vi "Read RawData.vi"(8 "error in (no error)":errorcluster, 9 "WCM_max_value":bool, 10 "# of scans":i32, 11 "Emulate in":refnum<class "Emulate.lvclass">) -> (0 "error out":errorcluster, 1 "Channel II":sgl[][](array[numeric]), 2 "Channel I":sgl[][](array[numeric]), 3 "Emulate out":refnum<class "Emulate.lvclass">, 4 "WCM_values":sgl[](array[numeric]))   [LabVIEW 2015, in "Emulate.lvclass"]
uses:
  Emulate.lvclass
  dependecies/globalVarII.vi
panel:
  out "Waveform Graph 2":i32[][](graph)
  out "Waveform Graph":i32[][](graph)
  in  "A":dbl=15000.0
  in  "pos":dbl=550.0 format="%#_13g"
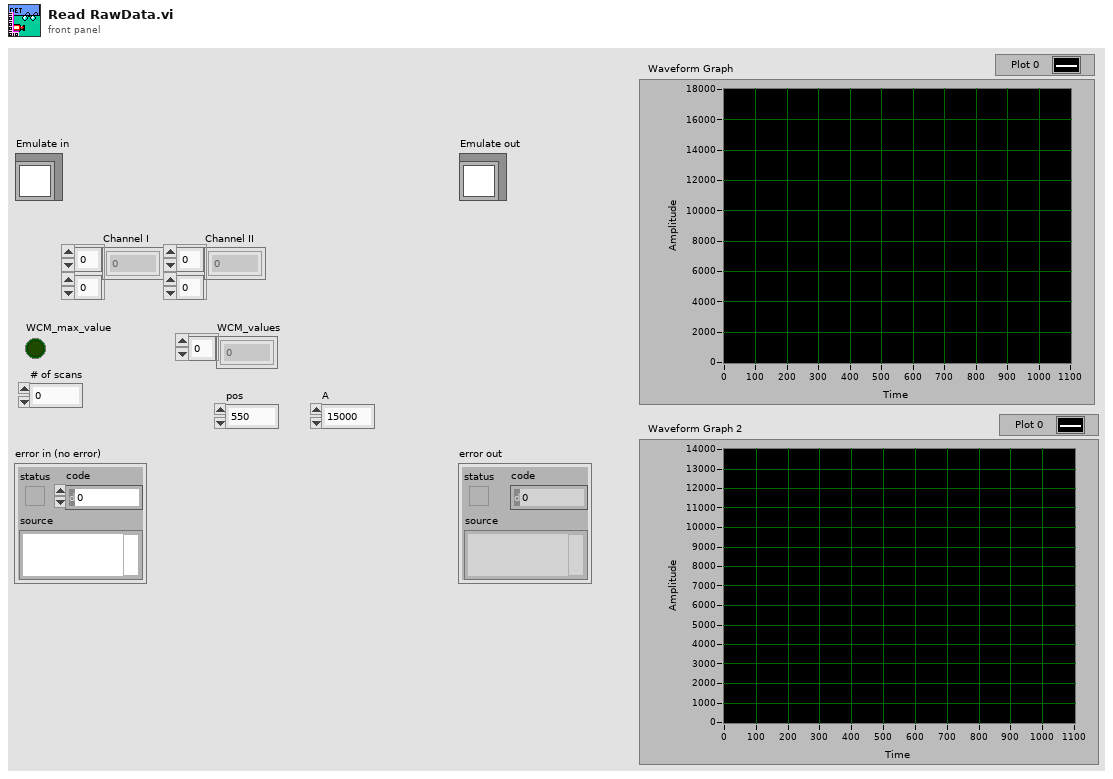
[diagram p1: front panel]
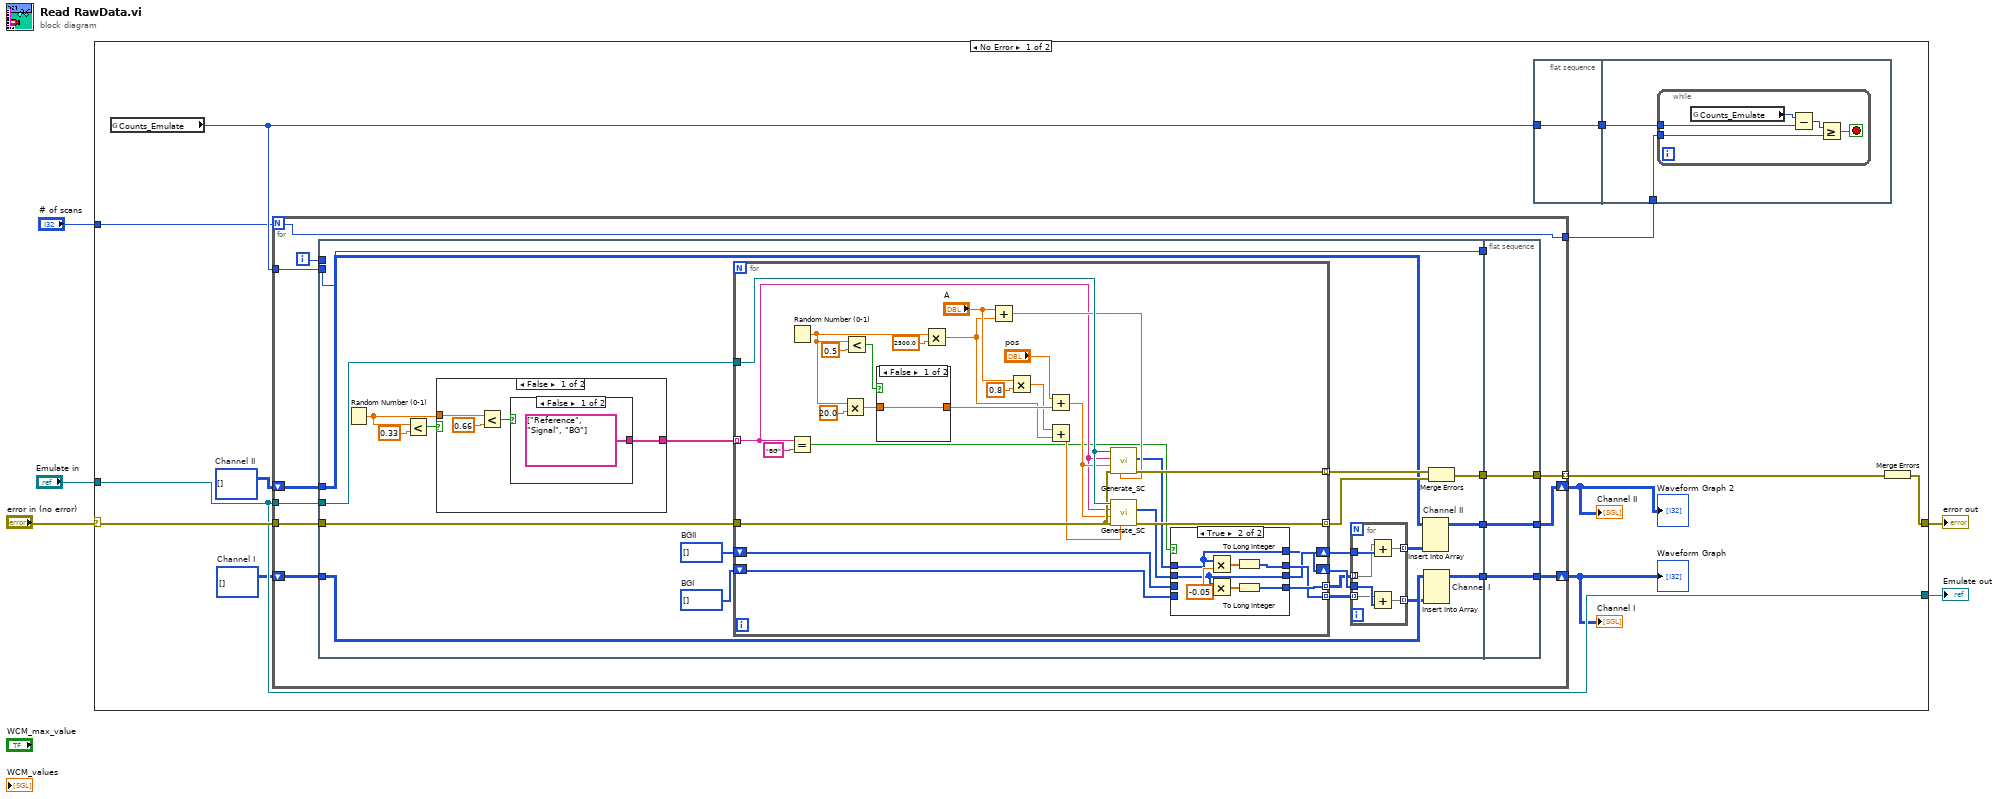
[diagram p0: block diagram]
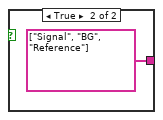
[diagram p2: hidden frame]
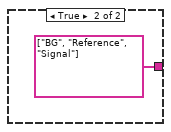
[diagram p3: hidden frame]
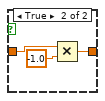
[diagram p5: hidden frame]
diagram:
  n1 = case shown="No Error" "error in (no error)" {
    selector: "error in (no error)" -> [w17 w124]
    tunnel: [w15 w124] -> w4
    tunnel: [w14 w123] -> w3
    tunnel: "Emulate in" -> [w14 w123]
    tunnel: "# of scans" -> [w9 _]
    frame No Error {
      w12 = i32[][] []  # Channel II
      w13 = i32[][] []  # Channel I
      n2 = global read "globalVarII.vi" "Counts_Emulate"() -> (w11:i64)
      n3 = for {
        N: w9 -> [w26]
        tunnel: w14 -> [w39]
        tunnel: w17 -> [w38]
        tunnel: [w37] -> w16 mode=indexing
        shift-right: [w36] -> w8
        shift-left: w13 -> [w35]
        shift-right: [w34] -> w7
        shift-left: w12 -> [w33]
        tunnel: w11 -> [w28]
        tunnel: [w26] -> w6
        i -> [w27]
        n4 = flat-sequence {
          tunnel: w39 -> [w57]
          tunnel: w38 -> [w56]
          tunnel: w35 -> [w51]
          tunnel: w33 -> [w49]
          tunnel: [w53] -> w32
          tunnel: [w52] -> w31
          tunnel: [w50] -> w30
          tunnel: [w48] -> w29
          tunnel: w28 -> [w48]
          tunnel: w27 -> [_]
          tunnel: [w120] -> w34
          tunnel: [w121] -> w36
          tunnel: [w122] -> w37
          tunnel: w32 -> [w122]
          tunnel: w31 -> [w121]
          tunnel: w30 -> [w120]
          tunnel: w29 -> [_]
          frame #0 {
            w47 = i32[] []  # BGII
            w46 = i32[] []  # BGI
            n5 = Random Number (0-1)() -> (number: 0 to 1=w58:dbl)
            n6 = Less?(x=w58, y=0.33) -> (x < y?=w59:bool)
            n7 = case shown="False" w59 {
              tunnel: [w68 string[] ["BG", "Reference", "Signal"] ("appended array")] -> w61
              tunnel: w58 -> [w71 _]
              frame False {
                n8 = Less?(x=w71, y=0.66) -> (x < y?=w69:bool)
                n9 = case shown="False" w69 {
                  tunnel: [string[] ["Reference", "Signal", "BG"] ("appended array") string[] ["Signal", "BG", "Reference"] ("appended array")] -> w68
                  frame False {
                  }
                  frame True {
                  }
                }
              }
              frame True {
              }
            }
            n10 = for {
              tunnel: w61 -> [w85] mode=indexing
              tunnel: w57 -> [w104]
              tunnel: w56 -> [w103]
              tunnel: [w102] -> w54 mode=indexing
              tunnel: [w101] -> w55 mode=indexing
              shift-right: [w80] -> w42
              shift-left: w47 -> [w79]
              shift-right: [w77] -> w45
              shift-left: w46 -> [w78]
              tunnel: [w82] -> w41 mode=indexing
              tunnel: [w81] -> w40 mode=indexing
              n11 = Random Number (0-1)() -> (number: 0 to 1=w93:dbl)
              n12 = Equal?(x=w85, y="BG") -> (x = y?=w83:bool)
              n13 = Multiply(x=w93, y=20.0) -> (x*y=w94:dbl)
              n14 = Less?(x=w93, y=0.5) -> (x < y?=w95:bool)
              n15 = case shown="False" w95 {
                tunnel: [w116 w117] -> w96
                tunnel: w94 -> [w116 w119]
                frame False {
                }
                frame True {
                  n16 = Multiply(x=w119, y=-1.0) -> (x*y=w117:dbl)
                }
              }
              n17 = Multiply(x=w93, y=2500.0) -> (x*y=w87:dbl)
              n18 = Add(x="A", y=w87) -> (x+y=w91:dbl)
              n19 = Multiply(x="A", y=0.8) -> (x*y=w88:dbl)
              n20 = Add(x="pos", y=w96) -> (x+y=w97:dbl)
              n21 = Add(x=w88, y=w87) -> (x+y=w86:dbl)
              n22 = call "Generate_SC.vi"("A"=w91, "error in (no error)"=w103, "pos"=w97, "Type of signal"=w85, "Emulate in"=w104) -> ("error out"=w101:errorcluster, "SC output"=w76:i32[])  [unwired: 4 in, 1 out]
              n23 = call "Generate_SC.vi"("A"=w86, "error in (no error)"=w103, "pos"=w97, "Type of signal"=w85, "Emulate in"=w104) -> ("error out"=w102:errorcluster, "SC output"=w75:i32[])  [unwired: 4 in, 1 out]
              n24 = case shown="True" w83 {
                tunnel: [w105 w111] -> w82
                tunnel: [w106 w112] -> w81
                tunnel: [w108 w109] -> w80
                tunnel: w79 -> [w108 _]
                tunnel: w78 -> [w107 _]
                tunnel: [w107 w110] -> w77
                tunnel: w76 -> [w106 w110]
                tunnel: w75 -> [w105 w109]
                frame False {
                }
                frame True {
                  w113 = -0.05
                  n25 = Multiply(x=w110, y=w113) -> (x*y=w115:dbl[])
                  n26 = Multiply(x=w109, y=w113) -> (x*y=w114:dbl[])
                  n27 = To Long Integer(number=w115) -> (32bit integer=w112:i32[])
                  n28 = To Long Integer(number=w114) -> (32bit integer=w111:i32[])
                }
              }
            }
            n29 = for {
              tunnel: w45 -> [w67]
              tunnel: [w66] -> w44 mode=indexing
              tunnel: [w65] -> w43 mode=indexing
              tunnel: w42 -> [w64]
              tunnel: w41 -> [w63] mode=indexing
              tunnel: w40 -> [w62] mode=indexing
              n30 = Add(x=w63, y=w64) -> (x+y=w65:i32[])
              n31 = Add(x=w62, y=w67) -> (x+y=w66:i32[])
            }
            n32 = Insert Into Array "Channel II"(array=w49, new element=w43) -> (w50:i32[][])  [unwired: 2 in]
            n33 = Insert Into Array "Channel I"(array=w51, new element=w44) -> (w52:i32[][])  [unwired: 2 in]
            n34 = Merge Errors(w55, w54) -> (w53:errorcluster)
          }
          frame #1 {
          }
        }
      }
      "Channel I" <- w8
      "Channel II" <- w7
      "Waveform Graph" <- w8
      "Waveform Graph 2" <- w7
      n35 = flat-sequence {
        tunnel: w11 -> [w18]
        tunnel: [w18] -> w10
        tunnel: w10 -> [w20]
        tunnel: w6 -> [w19]
        frame #0 {
        }
        frame #1 {
          n36 = while {
            tunnel: w20 -> [w23]
            tunnel: w19 -> [w21]
            stop <- w25 stop-if-true
            n37 = global read "globalVarII.vi" "Counts_Emulate"() -> (w24:i64)
            n38 = Subtract(x=w24, y=w23) -> (x-y=w22:i64)
            n39 = Greater Or Equal?(x=w22, y=w21) -> (x >= y?=w25:bool)
          }
        }
      }
      n40 = Merge Errors(w16) -> (w15:errorcluster)
    }
    frame Error {
    }
  }
  "error out" <- w4
  "Emulate out" <- w3
